vi "get Last Time.vi"(11 "Motion in":refnum<class "Motion.lvclass">) -> (3 "Last Time":dbl format="%_19f")   [LabVIEW 2015, in "Motion.lvclass"]
uses:
  Motion.lvclass
  Motion.lvclass/Motion.ctl
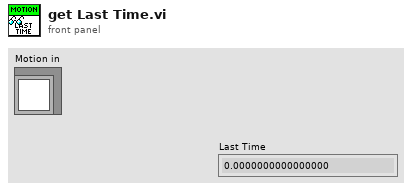
[diagram p1: front panel]
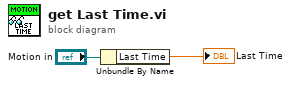
[diagram p0: block diagram]
diagram:
  n1 = Unbundle By Name("Motion in") -> ("Last Time"=→"Last Time":dbl)
